vi "to string.vi"(8 "error in":errorcluster, 11 "fixed channel configuration in":refnum<class "DAQmx Watchdog configuration.lvclass">) -> (0 "error out":errorcluster, 1 "data":string, 2 "version":string, 3 "fixed channel configuration out":refnum<class "DAQmx Watchdog configuration.lvclass">)   [LabVIEW 2014, in "DAQmx Watchdog configuration.lvclass"]
doc: "Provides an interface for saving a module configuration to a file or other serialized data source. It is recommended that all children of this class store data in two sets--data required for its own initialization, and any data required for parent initialization--and that each implementation uses the <b>Call Parent Method</b> primitive to serialize parent information.\nNI Tag Bus Module Framework 1.0.3.43\nNI Systems Engineering"
uses:
  DAQmx Watchdog configuration.lvclass
  <vilib>/NI/DCAF/Tag Editor Core/control module/configuration/control module configuration.lvclass
  <vilib>/NI/Configuration Framework/serializable configuration/NISE_CEF_serializable configuration.lvclass
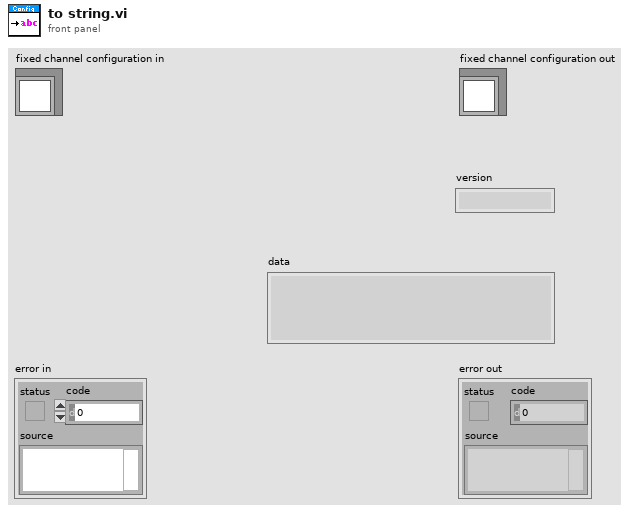
[diagram p1: front panel]
types:
  T1 = cluster{"physical channel":tag, "expiration state":dbl, "output type":i32}[]
  T2 = cluster{"physical channel(s)":tag, "expiration state":i32}[]
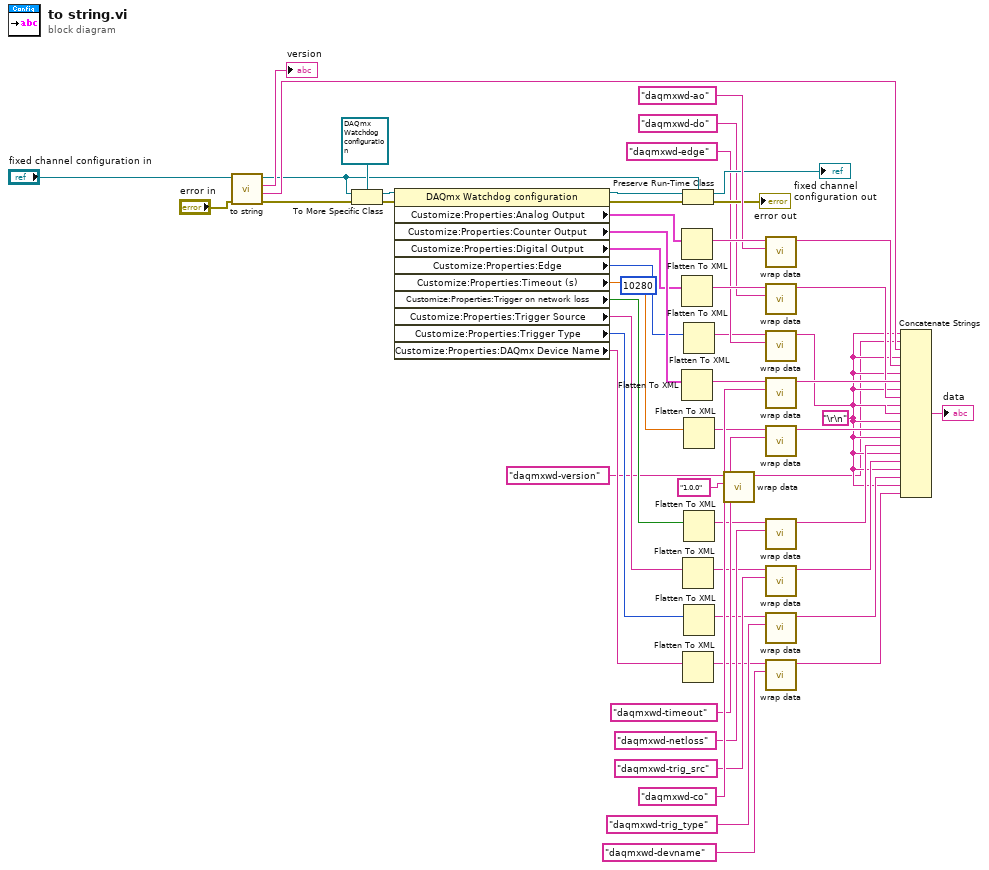
[diagram p0: block diagram]
diagram:
  (unwired) 10280 ("Edge")
  w4 = "\r\n"
  n1 = call-parent "to string.vi"("error in"="error in", "fixed channel configuration in"="fixed channel configuration in") -> ("error out"=w45:errorcluster, "data"=w52:string, "version"=→"version":string, "fixed channel configuration out"=w5:refnum<class "DAQmx Watchdog configuration.lvclass">)  [unwired: 6 in]
  n2 = To More Specific Class(target class=refnum<class "DAQmx Watchdog configuration.lvclass"> refnum, reference=w5, error in=w45) -> (specific class reference=w47:refnum<class "DAQmx Watchdog configuration.lvclass">, error out=w46:errorcluster)
  n3 = property class="DAQmx Watchdog configuration"(reference=w47, error in=w46) -> (reference out=w44:refnum<class "DAQmx Watchdog configuration.lvclass">, error out=w39:errorcluster, "Customize:Properties:Analog Output"=w41:T1, "Customize:Properties:Counter Output"=w35:T2, "Customize:Properties:Digital Output"=w31:T2, "Customize:Properties:Edge"=w27:i32, "Customize:Properties:Timeout (s)"=w23:dbl, "Customize:Properties:Trigger on network loss"=w20:bool, "Customize:Properties:Trigger Source"=w15:tag, "Customize:Properties:Trigger Type"=w10:i32, "Customize:Properties:DAQmx Device Name"=w6:tag)
  n4 = Flatten To XML(anything=w41) -> (xml string=w50:string)
  n5 = Flatten To XML(anything=w31) -> (xml string=w33:string)
  n6 = Flatten To XML(anything=w35) -> (xml string=w36:string)
  n7 = Preserve Run-Time Class(object in=w44, error in=w39, 2:w5) -> (object out=→"fixed channel configuration out":refnum<class "DAQmx Watchdog configuration.lvclass">, error out=→"error out":errorcluster)
  n8 = Flatten To XML(anything=w15) -> (xml string=w16:string)
  n9 = Flatten To XML(anything=w6) -> (xml string=w8:string)
  n10 = Flatten To XML(anything=w27) -> (xml string=w28:string)
  n11 = Flatten To XML(anything=w23) -> (xml string=w25:string)
  n12 = Flatten To XML(anything=w20) -> (xml string=w21:string)
  n13 = Flatten To XML(anything=w10) -> (xml string=w13:string)
  n14 = call <vilib>:"wrap data.vi"("identifier"="1.0.0", "data to wrap"="daqmxwd-version") -> ("wrapped data"=w3:string)  [unwired: 9 in]
  n15 = call <vilib>:"wrap data.vi"("identifier"="daqmxwd-ao", "data to wrap"=w50) -> ("wrapped data"=w40:string)  [unwired: 9 in]
  n16 = call <vilib>:"wrap data.vi"("identifier"="daqmxwd-do", "data to wrap"=w33) -> ("wrapped data"=w30:string)  [unwired: 9 in]
  n17 = call <vilib>:"wrap data.vi"("identifier"="daqmxwd-edge", "data to wrap"=w28) -> ("wrapped data"=w26:string)  [unwired: 9 in]
  n18 = call <vilib>:"wrap data.vi"("identifier"="daqmxwd-co", "data to wrap"=w36) -> ("wrapped data"=w34:string)  [unwired: 9 in]
  n19 = call <vilib>:"wrap data.vi"("identifier"="daqmxwd-timeout", "data to wrap"=w25) -> ("wrapped data"=w22:string)  [unwired: 9 in]
  n20 = call <vilib>:"wrap data.vi"("identifier"="daqmxwd-netloss", "data to wrap"=w21) -> ("wrapped data"=w19:string)  [unwired: 9 in]
  n21 = call <vilib>:"wrap data.vi"("identifier"="daqmxwd-trig_src", "data to wrap"=w16) -> ("wrapped data"=w14:string)  [unwired: 9 in]
  n22 = call <vilib>:"wrap data.vi"("identifier"="daqmxwd-trig_type", "data to wrap"=w13) -> ("wrapped data"=w11:string)  [unwired: 9 in]
  n23 = call <vilib>:"wrap data.vi"("identifier"="daqmxwd-devname", "data to wrap"=w8) -> ("wrapped data"=w7:string)  [unwired: 9 in]
  n24 = Concatenate Strings(w4, w3, w52, w4, w40, w4, w34, w4, w30, w4, w26, w4, w22, w4, w19, w4, w14, w4, w11, w4, w7) -> (→"data":string)
